vi "parseMassdata.vi"(11 "Arguments":string) -> (3 "unpacked source data 1":waveform(dbl)(graph))   [LabVIEW 2017, in "massdataInlvlibp.lvlib"]
uses:
  massdataInlvlibp.lvlib
  d89c5cbc-74be-4702-a14c-3c4deee51a53.vi
  addons/MassData-Parameter/_support/FGV-MassData(lvlibp).vi
  <userlib>/_NEVSTOP/Communicable State Machine(CSM)/_Shared/CSM Shared.lvlib
panel:
  out "Arg Token 2":string
  out "CSM Argument(as <massdata>) 2":string
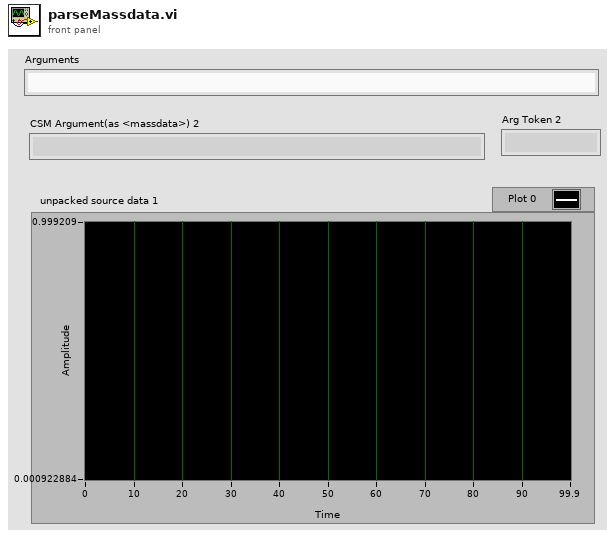
[diagram p1: front panel]
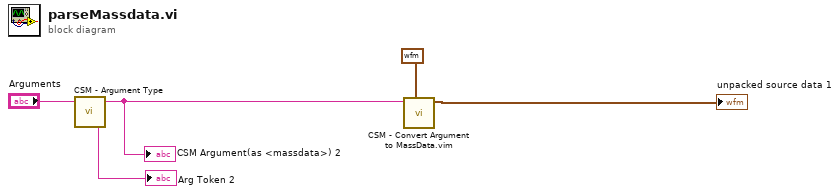
[diagram p0: block diagram]
diagram:
  n1 = call <userlib>:"CSM - Argument Type.vi"("Arguments"="Arguments") -> ("Argument Type"=→"Arg Token 2":string, "Arguments (Dup)"=w4:string)  [unwired: 3 in]
  "CSM Argument(as <massdata>) 2" <- w4
  n2 = call "CSM - Convert Argument to MassData.vim"("Type"=waveform(dbl) {"t0"=timestamp(0 s since 1904-01-01), "dt"=1.0, "Y"=[]} ("Waveform"), "MassData Argument"=w4) -> ("Data"=→"unpacked source data 1":waveform(dbl))  [unwired: 6 in, 1 out]
